vi "Normal.vi"(11 "Triangle":T2={"Point 1"={"x"=0.0, "y"=0.0, "z"=0.0}, "Point 2"={"x"=0.0, "y"=0.0, "z"=0.0}, "Point 3"={"x"=0.0, "y"=0.0, "z"=0.0}, "Fill Colour"=12517256}) -> (3 "Normal":T1)   [LabVIEW 2022 SP3, in "3D.lvlib"]
uses:
  3D.lvlib
  Triangle 3D.ctl
  Vector 3D.ctl
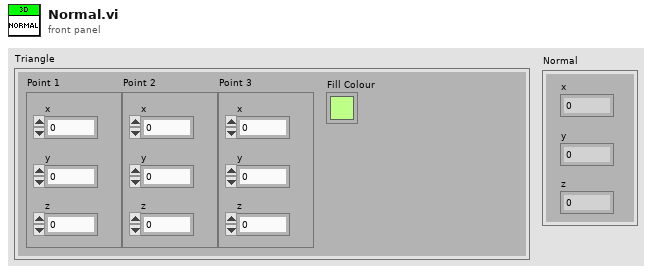
[diagram p1: front panel]
types:
  T1 = typedef "3D.lvlib/Vector 3D.ctl" = cluster{"x":sgl, "y":sgl, "z":sgl}
  T2 = typedef "3D.lvlib/Triangle 3D.ctl" = cluster{"Point 1":T1, "Point 2":T1, "Point 3":T1, "Fill Colour":u32}
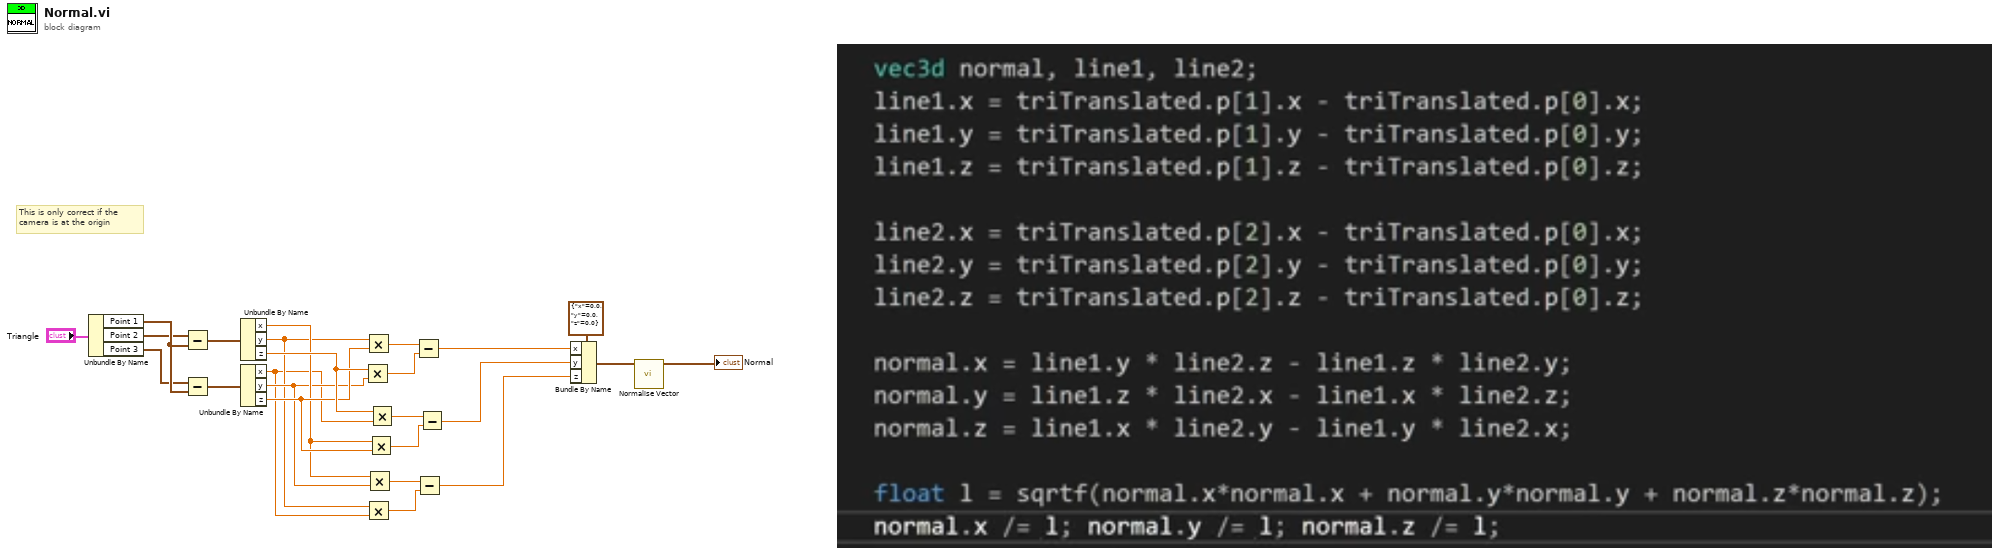
[diagram p0: block diagram]
diagram:
  # "This is only correct if the camera is at the origin"
  n1 = Unbundle By Name("Triangle") -> ("Point 1"=w3:T1, "Point 2"=w2:T1, "Point 3"=w1:T1)
  n2 = Subtract(x=w2, y=w3) -> (x-y=w22:T1)
  n3 = Subtract(x=w1, y=w3) -> (x-y=w21:T1)
  n4 = Unbundle By Name(w22) -> ("x"=w9:sgl, "y"=w7:sgl, "z"=w11:sgl)
  n5 = Unbundle By Name(w21) -> ("x"=w6:sgl, "y"=w8:sgl, "z"=w10:sgl)
  n6 = Multiply(x=w11, y=w8) -> (x*y=w19:sgl)
  n7 = Multiply(x=w7, y=w10) -> (x*y=w20:sgl)
  n8 = Multiply(x=w7, y=w6) -> (x*y=w14:sgl)
  n9 = Multiply(x=w9, y=w8) -> (x*y=w15:sgl)
  n10 = Multiply(x=w9, y=w10) -> (x*y=w17:sgl)
  n11 = Multiply(x=w11, y=w6) -> (x*y=w16:sgl)
  n12 = Subtract(x=w20, y=w19) -> (x-y=w18:sgl)
  n13 = Subtract(x=w15, y=w14) -> (x-y=w12:sgl)
  n14 = Subtract(x=w16, y=w17) -> (x-y=w13:sgl)
  n15 = Bundle By Name(cluster=T1 {"x"=0.0, "y"=0.0, "z"=0.0} ("Normal"), "x"=w18, "y"=w13, "z"=w12) -> (w5:T1)
  n16 = call "Normalise Vector.vi"("Vector 3D"=w5) -> ("Vector 3D Normalised"=→"Normal":T1)  [unwired: 10 in]
